vi "Test EXE.vi"() -> ()   [LabVIEW 2020]
panel:
  out "Current VI's Path (+ Relative)":path
  out "Application Directory":path
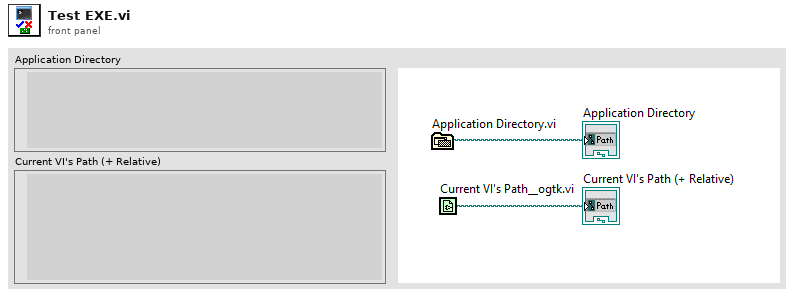
[diagram p1: front panel]
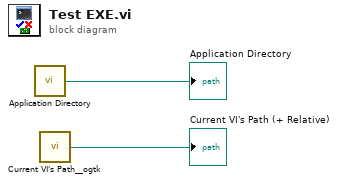
[diagram p0: block diagram]
diagram:
  n1 = call <vilib>:"Application Directory.vi"() -> ("Application Directory"=→"Application Directory":path)
  n2 = call <userlib>:"Current VI's Path__ogtk.vi"() -> ("Current VI's Path (+ Relative)"=→"Current VI's Path (+ Relative)":path)  [unwired: 1 in]
